vi "KVMap-To String.vi"(7 "string":string=":", 11 "Cluster":cluster{string[], string[]}) -> (3 "value":string)   [LabVIEW 2012]
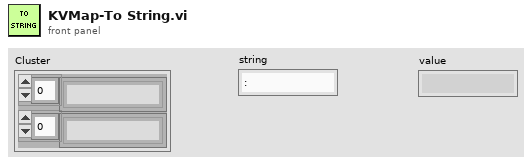
[diagram p1: front panel]
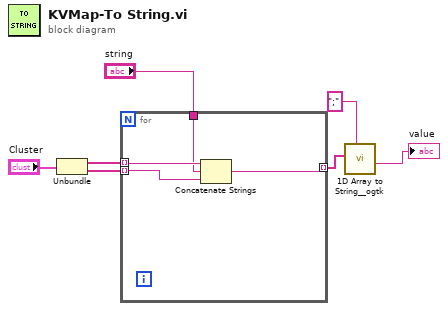
[diagram p0: block diagram]
diagram:
  n1 = Unbundle("Cluster") -> (w6:string[], w5:string[])
  n2 = for {
    tunnel: w6 -> [w11] mode=indexing
    tunnel: w5 -> [w10] mode=indexing
    tunnel: [w9] -> w4 mode=indexing
    tunnel: "string" -> [w8]
    n3 = Concatenate Strings(w11, w8, w10) -> (w9:string)
  }
  n4 = call <userlib>:"1D Array to String__ogtk.vi"("delimiter (Tab)"=";", "Array of Strings"=w4) -> ("delimited string"=→"value":string)  [unwired: 9 in]
